vi "1.PROYECTO_FINAL_ESTACIONAMIENTO.vi"() -> ()   [LabVIEW 2025]
uses:
  <vilib>/userDefined/High Color/IMAQdx.ctl
  <vilib>/httpClient/LabVIEWHTTPClient.lvlib
  <vilib>/vision/driver/NI_Vision_Acquisition_Software.lvlib
  <vilib>/vision/NI_Vision_Development_Module.lvlib
panel:
  in  "PAGAR":bool
  out "Total a pagar":string
  out "Tiempo":string
  out "ID TICKET":string
  out "LED1":bool
  out "LED3":bool
  out "LED2":bool
  out "?":string
  out "?":string
  out "LED ticket":bool
  in  "QR_boton":bool
  out "Cámara Estacionamiento":T1(plugin-control)
  out "Camara Qr":T1(plugin-control)
  in  "stop":bool
  out "QR":T1(plugin-control)
  # "ID TICKET"
  # "TIEMPO:"
  # "TOTAL A PAGAR:"
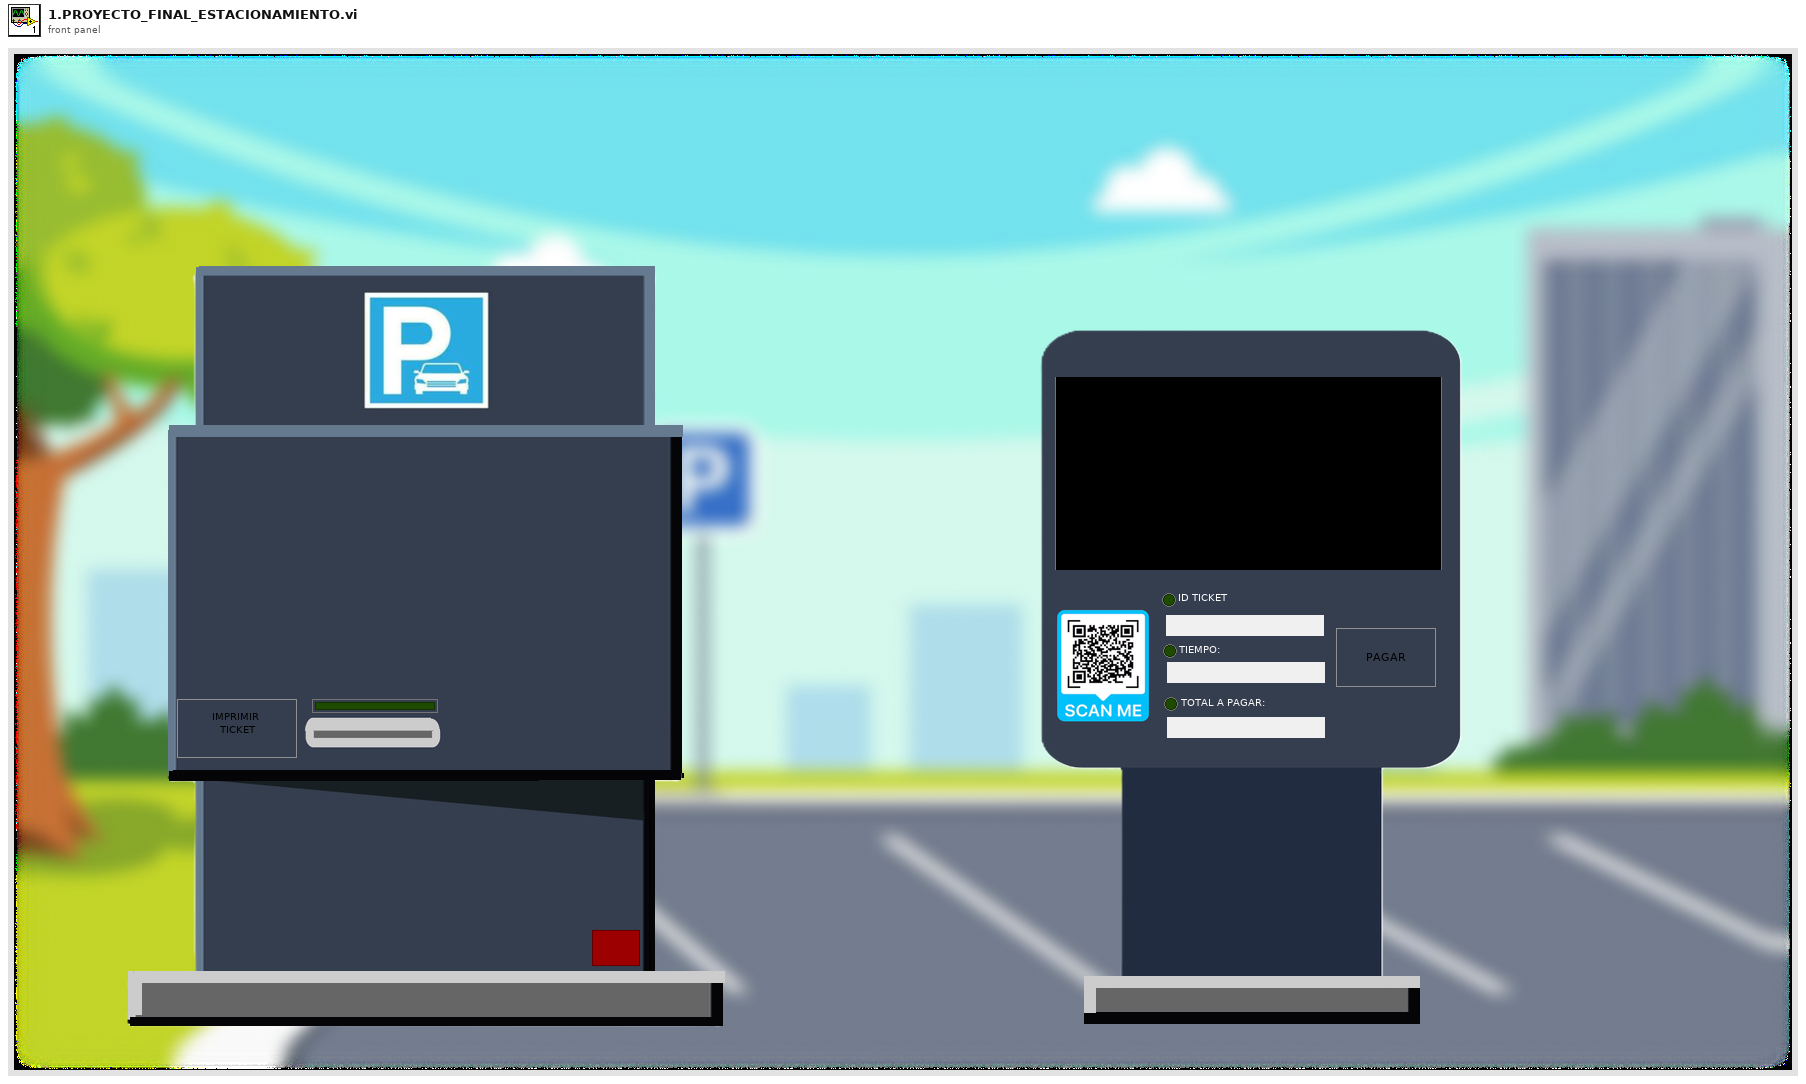
[diagram p1: front panel]
types:
  T1 = typedef "IMAQ Image.ctl" = refnum<image>
  T2 = typedef "Image Type" = u32
  T3 = typedef "IMAQdx.ctl" = refnum<k21>
  T4 = typedef "LabVIEWHTTPClient.lvlib/ClientHandle.ctl" = refnum<k1>
  T5 = typedef "QR Code Report.ctl" = cluster{"Found?":bool, "Data":string, "Bounding Box":cluster{"x":sgl, "y":sgl}[], "Errors Corrected":u32, "Dimensions (Rows/Cols)":u32, "Version":u32, "QR Model":T6, "Stream Mode":T7, "Barcode Polarity":T8, "Mirrored?":bool, "Append Stream Position":u32, "Size of Append Stream":u32, "First EAN-128 ID":i32, "First Alternate Language ID":i32, "Append Stream ID":u32, "Minimum Edge Strength":u32, "Demodulation Mode":T9, "Cell Sample Size":T10, "Cell Filter Mode":T11}
  T6 = typedef "QR Code Model Type.ctl" = i32
  T7 = typedef "QR Code Stream Mode Type.ctl" = i32
  T8 = typedef "Data Matrix Polarity.ctl" = i32
  T9 = typedef "Demodulation Mode.ctl" = i32
  T10 = typedef "Cell Sample Size.ctl" = i32
  T11 = typedef "Cell Filter Mode.ctl" = i32
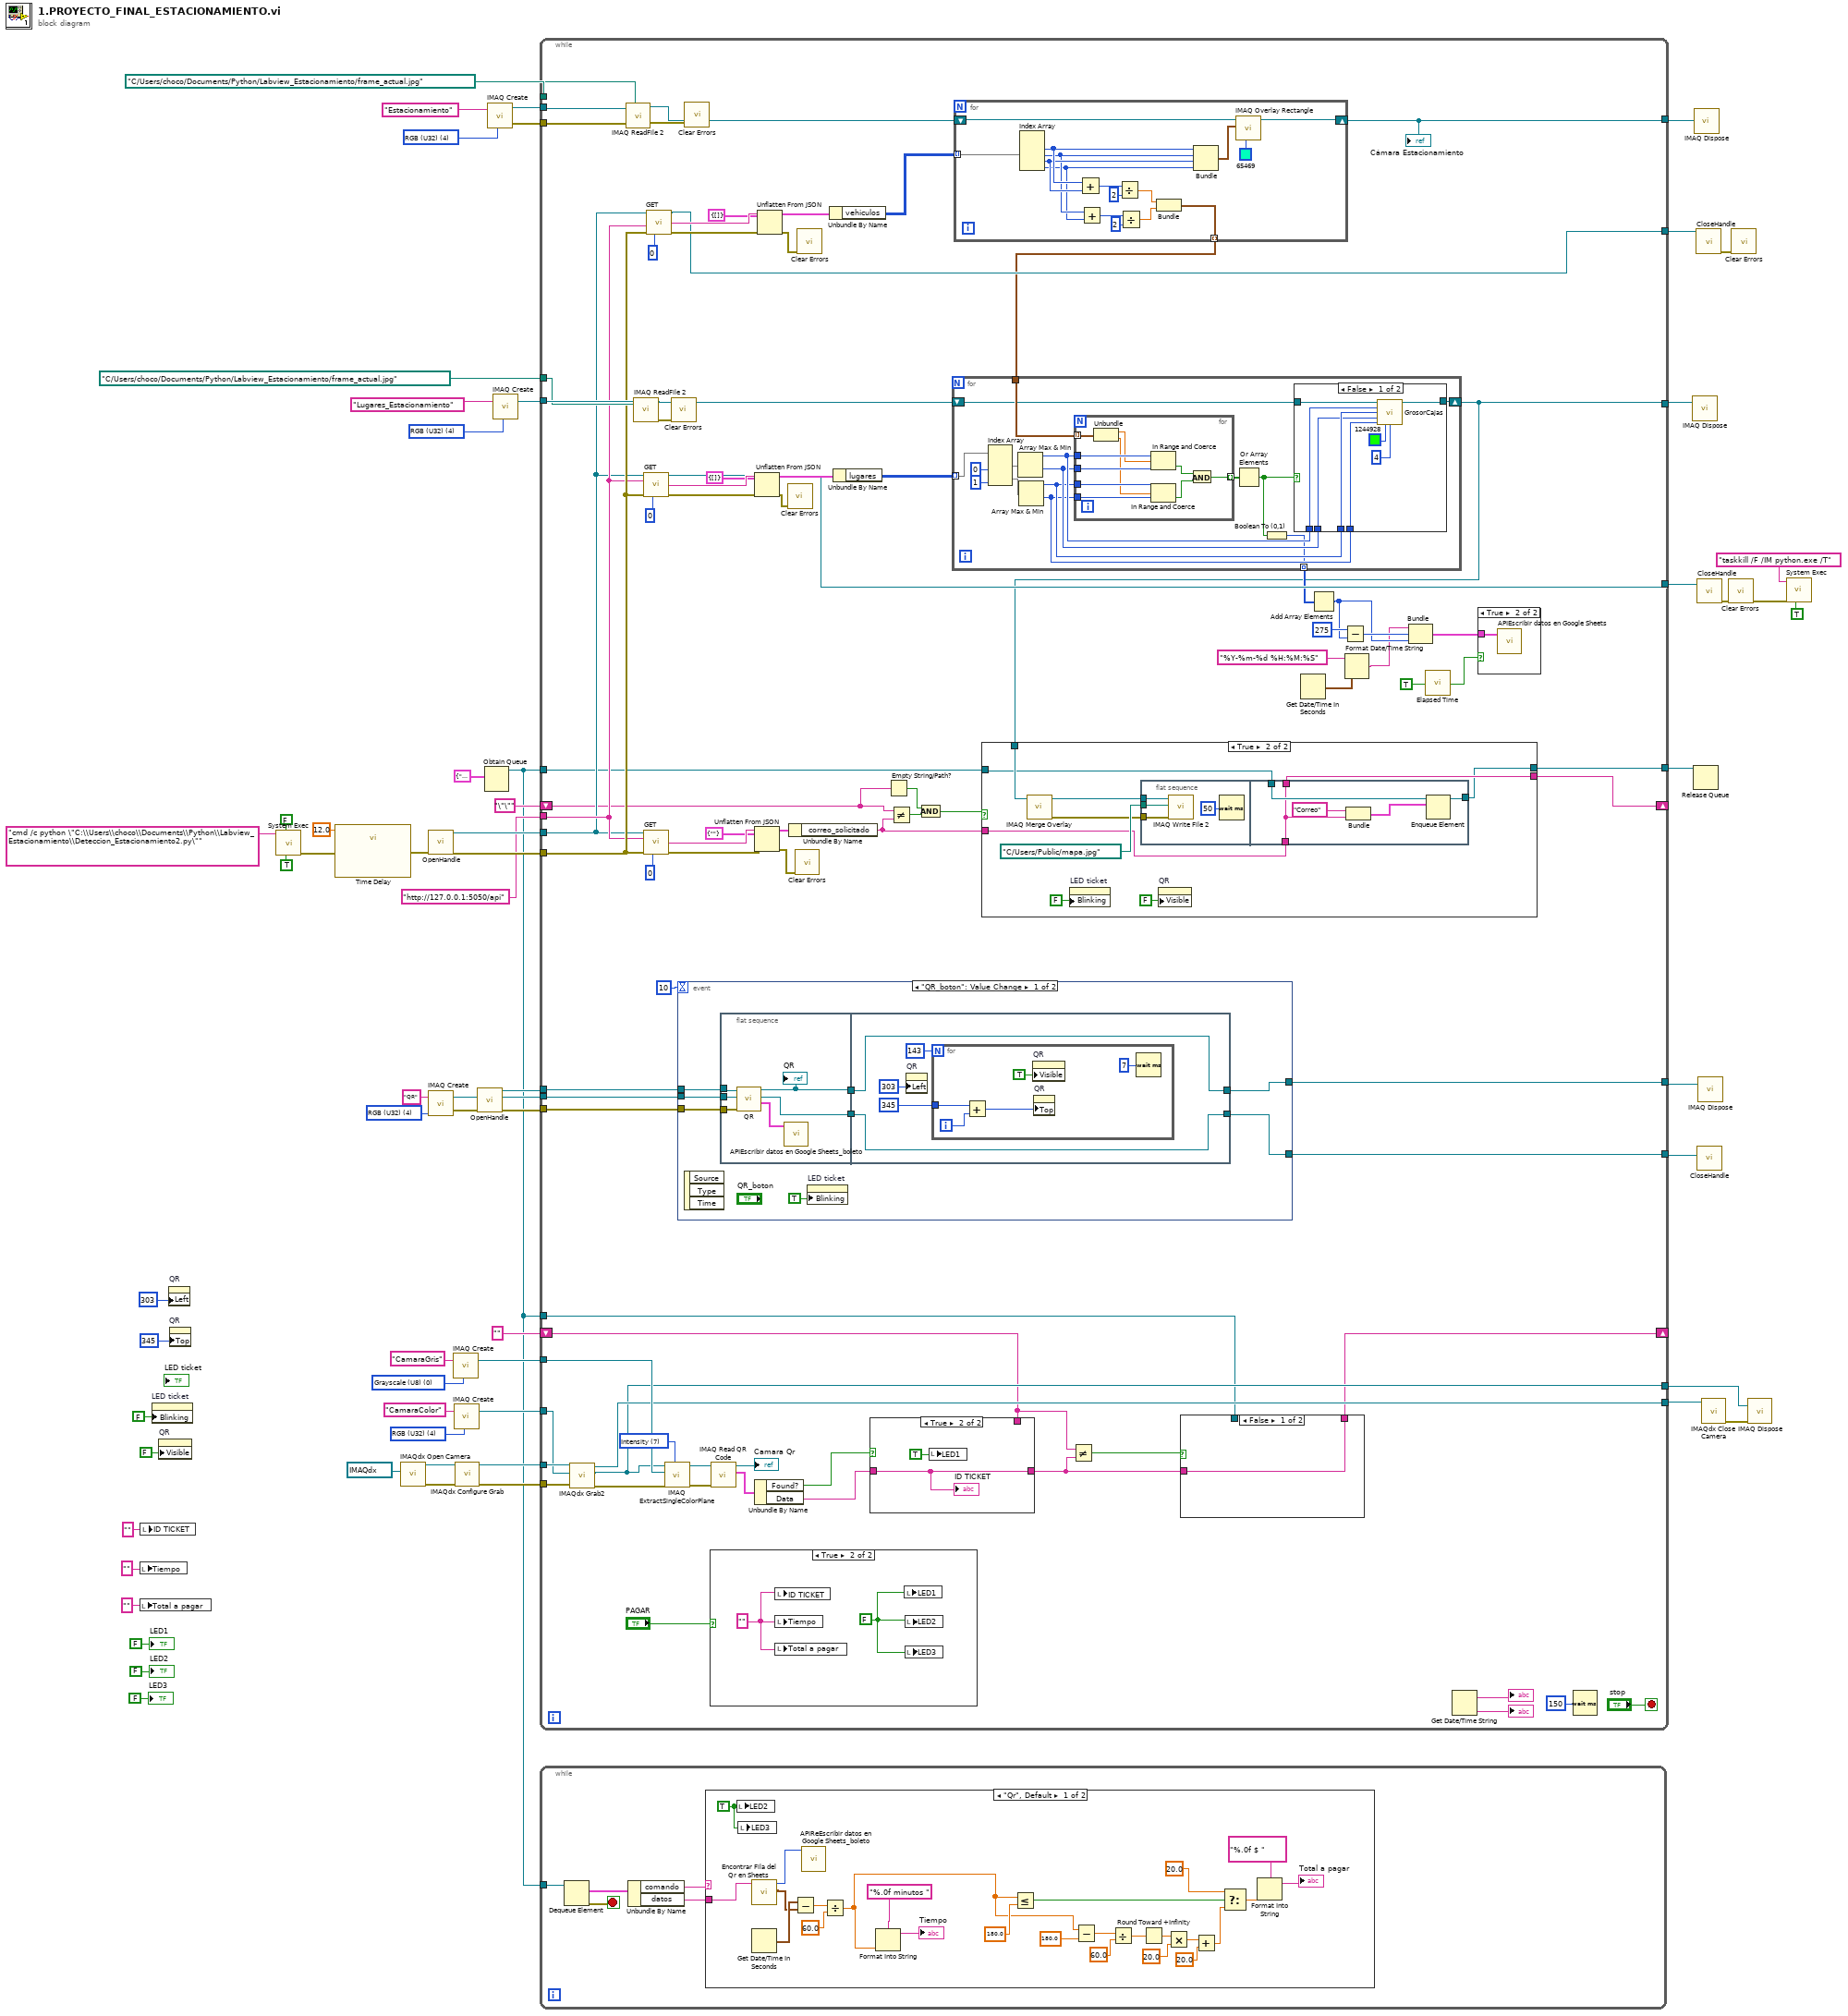
[diagram p0: block diagram]
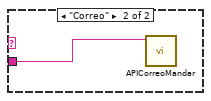
[diagram p2: hidden frame]
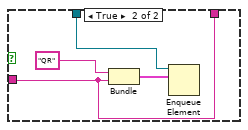
[diagram p4: hidden frame]
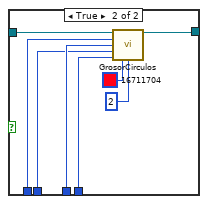
[diagram p7: hidden frame]
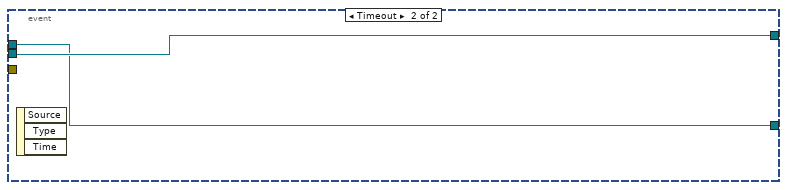
[diagram p9: hidden frame]
diagram:
  w21 = T2 0 items=["Grayscale (U8)", "Grayscale (I16)", "Grayscale (SGL)", "Complex (CSG)", "RGB (U32)", "HSL (U32)", "RGB (U64)", "Grayscale (U16)"] ("Image Type")
  w27 = T2 4 items=["Grayscale (U8)", "Grayscale (I16)", "Grayscale (SGL)", "Complex (CSG)", "RGB (U32)", "HSL (U32)", "RGB (U64)", "Grayscale (U16)"] ("Image Type")
  w38 = T2 4 items=["Grayscale (U8)", "Grayscale (I16)", "Grayscale (SGL)", "Complex (CSG)", "RGB (U32)", "HSL (U32)", "RGB (U64)", "Grayscale (U16)"] ("Image Type")
  w49 = T2 4 items=["Grayscale (U8)", "Grayscale (I16)", "Grayscale (SGL)", "Complex (CSG)", "RGB (U32)", "HSL (U32)", "RGB (U64)", "Grayscale (U16)"] ("Image Type")
  w62 = T2 4 items=["Grayscale (U8)", "Grayscale (I16)", "Grayscale (SGL)", "Complex (CSG)", "RGB (U32)", "HSL (U32)", "RGB (U64)", "Grayscale (U16)"] ("Image Type")
  n1 = local write "Tiempo"("" ("Tiempo")) -> ()
  n2 = local write "Total a pagar"("" ("Total a pagar")) -> ()
  n3 = local write "ID TICKET"("" ("ID TICKET")) -> ()
  n4 = property on="LED ticket" class="Bool (strict)"("Blinking"=FALSE) -> ()  [unwired: 2 in, 2 out]
  n5 = property on="QR" class="ImageControl"("Visible"=FALSE) -> ()  [unwired: 2 in, 2 out]
  n6 = property on="QR" class="ImageControl"("Left"=303 ("Position:Left")) -> ()  [unwired: 2 in, 2 out]
  n7 = property on="QR" class="ImageControl"("Top"=345 ("Position:Top")) -> ()  [unwired: 2 in, 2 out]
  n8 = call <vilib>:"System Exec.vi"("run minimized? (F)"=TRUE, "wait until completion? (T)"=FALSE, "command line"="cmd /c python \"C:\\Users\\choco\\Documents\\Python\\Labview_Estacionamiento\\Deteccion_Estacionamiento2.py\"") -> ("error out"=w58:errorcluster)  [unwired: 5 in, 3 out]
  n9 = call "Time Delay"("error in (no error)"=w58, "Delay Time (s)"=12.0) -> ("error out"=w55:errorcluster)  [unwired: 9 in]
  n10 = call <vilib>:"IMAQdx Open Camera.vi"("Session In"=T3 "cam0") -> ("error out"=w24:errorcluster, "Session Out"=w25:T3)  [unwired: 9 in]
  n11 = call <vilib>:"OpenHandle.vi"("error in (no error)"=w55) -> ("client handle out"=w31:T4, "error out"=w32:errorcluster)  [unwired: 13 in]
  n12 = call "IMAQ Create"("Image Name"="QR", "Image Type"=w49) -> ("New Image"=w48:T1, "error out"=w45:errorcluster)  [unwired: 3 in]
  n13 = call "IMAQ Create"("Image Name"="CamaraGris", "Image Type"=w21) -> ("New Image"=w17:T1)  [unwired: 3 in, 1 out]
  n14 = call "IMAQ Create"("Image Name"="CamaraColor", "Image Type"=w27) -> ("New Image"=w18:T1)  [unwired: 3 in, 1 out]
  n15 = call <vilib>:"IMAQdx Configure Grab.vi"("error in"=w24, "Session In"=w25) -> ("error out"=w19:errorcluster, "Session Out"=w20:T3)  [unwired: 8 in]
  n16 = call <vilib>:"OpenHandle.vi"("error in (no error)"=w45) -> ("client handle out"=w46:T4, "error out"=w44:errorcluster)  [unwired: 13 in]
  n17 = Obtain Queue(element data type=cluster{"comando":string, "datos":string} {"comando"="", "datos"=""}) -> (queue out=w11:refnum<queue>)  [unwired: 4 in, 2 out]
  n18 = call "IMAQ Create"("Image Name"="Estacionamiento", "Image Type"=w62) -> ("New Image"=w61:T1, "error out"=w54:errorcluster)  [unwired: 3 in]
  n19 = call "IMAQ Create"("Image Name"="Lugares_Estacionamiento", "Image Type"=w38) -> ("New Image"=w37:T1)  [unwired: 3 in, 1 out]
  n20 = while {
    tunnel: path "C:/Users/choco/Documents/Python/Labview_Estacionamiento/frame_actual.jpg" ("path to JPEG file") -> [w147]
    tunnel: w61 -> [w148]
    tunnel: w54 -> [w145]
    tunnel: [w142] -> w51
    tunnel: w44 -> [w141]
    tunnel: w48 -> [w140]
    tunnel: [w139] -> w47
    tunnel: w46 -> [w138]
    tunnel: [w128] -> w43
    tunnel: [w122] -> w40
    tunnel: w37 -> [w117]
    tunnel: path "C:/Users/choco/Documents/Python/Labview_Estacionamiento/frame_actual.jpg" ("path to JPEG file 2") -> [w116]
    tunnel: [w114] -> w35
    tunnel: [w94] -> w34
    tunnel: w32 -> [w101]
    tunnel: w31 -> [w99]
    tunnel: "http://127.0.0.1:5050/api" ("url") -> [w100]
    shift-right: [w93] -> _
    shift-left: "\"\"" -> [w92]
    tunnel: w11 -> [w90]
    tunnel: w20 -> [w85]
    tunnel: w19 -> [w84]
    tunnel: w18 -> [w83]
    tunnel: w17 -> [w82]
    tunnel: [w81] -> w16
    tunnel: [w80] -> w15
    tunnel: [w79] -> w14
    shift-right: [w73] -> _
    shift-left: "" -> [w68]
    tunnel: w11 -> [w70]
    stop <- "stop" stop-if-true
    w86 = 7 items=["Red", "Green", "Blue", "Hue", "Saturation", "Luminance", "Value", "Intensity"] ("Color Plane")
    n21 = call <vilib>:"IMAQdx Grab2.vi"("error in"=w84, "Image In"=w83, "Session In"=w85) -> ("error out"=w87:errorcluster, "Image Out"=w80:T1, "Session Out"=w81:T3)  [unwired: 5 in, 1 out]
    n22 = call "IMAQ ReadFile 2"("File Path"=w147, "error in (no error)"=w145, "Image"=w148) -> ("error out"=w146:errorcluster, "Image Out"=w119:T1)  [unwired: 4 in, 3 out]
    n23 = call "IMAQ ReadFile 2"("File Path"=w116, "Image"=w117) -> ("error out"=w118:errorcluster, "Image Out"=w115:T1)  [unwired: 5 in, 3 out]
    n24 = call <vilib>:"GET.vi"("client handle"=w99, "url"=w100, "error in (no error)"=w101, "timeout (10000)"=0) -> ("client handle out"=w122:T4, "body"=w127:string, "error out"=w126:errorcluster)  [unwired: 8 in, 1 out]
    n25 = call <vilib>:"GET.vi"("client handle"=w99, "url"=w100, "error in (no error)"=w101, "timeout (10000)"=0) -> ("body"=w105:string, "error out"=w104:errorcluster)  [unwired: 8 in, 2 out]
    n26 = call <vilib>:"GET.vi"("client handle"=w99, "url"=w100, "error in (no error)"=w101, "timeout (10000)"=0) -> ("client handle out"=w128:T4, "body"=w136:string, "error out"=w135:errorcluster)  [unwired: 8 in, 1 out]
    n27 = call "IMAQ ExtractSingleColorPlane"("Color Plane"=w86, "error in (no error)"=w87, "Image Dst"=w82, "Image Src"=w80) -> ("error out"=w76:errorcluster, "Image Dst Out"=w77:T1)  [unwired: 6 in]
    n28 = call <vilib>:"Clear Errors.vi"("error in (no error)"=w118) -> ()  [unwired: 5 in, 2 out]
    n29 = event shown="[0] \"QR_boton\": Value Change" {
      selector: _ -> [_ _]
      dyn-events: _ -> [_ _]
      timeout: 10 -> [_ _]
      tunnel: [w242 w264] -> w142
      tunnel: w141 -> [w246 _]
      tunnel: w140 -> [w245 w264]
      tunnel: [w243 w263] -> w139
      tunnel: w138 -> [w244 w263]
      event "QR_boton": Value Change {
        n30 = event-data() -> ()  [unwired: 1 in, 3 out]
        n31 = flat-sequence {
          tunnel: w246 -> [w252]
          tunnel: w245 -> [w251]
          tunnel: w244 -> [w250]
          tunnel: [w249] -> w241
          tunnel: [w248] -> w240
          tunnel: [w257] -> w242
          tunnel: [w256] -> w243
          tunnel: w241 -> [w256]
          tunnel: w240 -> [w257]
          frame #0 {
            n32 = call "QR.vi"("error in (no error)"=w252, "Image"=w251, "client handle"=w250) -> ("value"=w247:cluster{"id":string, "hora_entrada":string}, "client handle out"=w249:T4, "QR Imagen"=w248:T1)  [unwired: 6 in]
            "QR" <- w248
            n33 = call "APIEscribir datos en Google Sheets_boleto.vi"("Cluster"=w247) -> ()  [unwired: 10 in]
          }
          frame #1 {
            n34 = property on="QR" class="ImageControl"("Left"=303 ("Position:Left")) -> ()  [unwired: 2 in, 2 out]
            n35 = for {
              N: 143 -> [_]
              tunnel: 345 ("Position:Top") -> [w259]
              i -> [w262]
              n36 = Add(x=w259, y=w262) -> (x+y=w261:i32)
              n37 = property on="QR" class="ImageControl"("Visible"=TRUE) -> ()  [unwired: 2 in, 2 out]
              n38 = property on="QR" class="ImageControl"("Top"=w261) -> ()  [unwired: 2 in, 2 out]
              n39 = Wait (ms)(milliseconds to wait=u32 7) -> ()  [unwired: 1 out]
            }
          }
        }
        n40 = property on="LED ticket" class="Bool (strict)"("Blinking"=TRUE) -> ()  [unwired: 2 in, 2 out]
      }
      event Timeout {
        n41 = event-data() -> ()  [unwired: 1 in, 3 out]
      }
    }
    n42 = call <vilib>:"Clear Errors.vi"("error in (no error)"=w146) -> ()  [unwired: 5 in, 2 out]
    n43 = case shown="True" "PAGAR" {
      frame False {
      }
      frame True {
        w150 = FALSE
        w151 = "" ("ID TICKET")
        n44 = local write "ID TICKET"(w151) -> ()
        n45 = local write "Tiempo"(w151) -> ()
        n46 = local write "Total a pagar"(w151) -> ()
        n47 = local write "LED1"(w150) -> ()
        n48 = local write "LED2"(w150) -> ()
        n49 = local write "LED3"(w150) -> ()
      }
    }
    n50 = call "IMAQ Read QR Code"("error in (no error)"=w76, "Image"=w77) -> ("QR Code Report"=w78:T5, "Image (duplicate)"=→"Camara Qr":T1)  [unwired: 6 in, 2 out]
    n51 = Unbundle By Name(w78) -> ("Found?"=w75:bool, "Data"=w74:string)
    n52 = Unflatten From JSON(JSON string=w127, type and defaults=cluster{"lugares":i32[][][]} {"lugares"=[]}, error in (no error)=w126) -> (value=w123:cluster{"lugares":i32[][][]}, error out=w71:errorcluster)  [unwired: 4 in]
    n53 = Unflatten From JSON(JSON string=w105, type and defaults=cluster{"correo_solicitado":string} {"correo_solicitado"=""}, error in (no error)=w104) -> (value=w98:cluster{"correo_solicitado":string}, error out=w69:errorcluster)  [unwired: 4 in]
    n54 = Unflatten From JSON(JSON string=w136, type and defaults=cluster{"vehiculos":i32[][]} {"vehiculos"=[]}, error in (no error)=w135) -> (value=w132:cluster{"vehiculos":i32[][]}, error out=w72:errorcluster)  [unwired: 4 in]
    n55 = call <vilib>:"Clear Errors.vi"("error in (no error)"=w71) -> ()  [unwired: 5 in, 2 out]
    n56 = Unbundle By Name(w98) -> ("correo_solicitado"=w91:string)
    n57 = call <vilib>:"Clear Errors.vi"("error in (no error)"=w69) -> ()  [unwired: 5 in, 2 out]
    n58 = call <vilib>:"Clear Errors.vi"("error in (no error)"=w72) -> ()  [unwired: 5 in, 2 out]
    n59 = Unbundle By Name(w132) -> ("vehiculos"=w131:i32[][])
    n60 = Unbundle By Name(w123) -> ("lugares"=w121:i32[][][])
    n61 = case shown="True" w75 {
      tunnel: w74 -> [_ w159]
      tunnel: [w157 w159] -> w67
      tunnel: w68 -> [w157 _]
      frame False {
      }
      frame True {
        n62 = local write "LED1"(TRUE ("LED1")) -> ()
        "ID TICKET" <- w159
      }
    }
    n63 = Empty String/Path?(string/path=w92) -> (empty?=w96:bool)
    n64 = Not Equal?(x=w92, y=w91) -> (x != y?=w97:bool)
    n65 = And(x=w96, y=w97) -> (x .and. y?=w95:bool)
    n66 = for {
      tunnel: w131 -> [w238] mode=indexing
      shift-right: [w236] -> w114
      shift-left: w119 -> [w234]
      tunnel: [w223] -> w120 mode=indexing
      n67 = Index Array(array=w238) -> (element #1=w233:i32, element #2=w227:i32, element #3=w232:i32, element #4=w226:i32)  [unwired: 4 in]
      n68 = Add(x=w233, y=w232) -> (x+y=w231:i32)
      n69 = Add(x=w227, y=w226) -> (x+y=w229:i32)
      n70 = Divide(x=w231, y=2) -> (x/y=w225:dbl)
      n71 = Divide(x=w229, y=2) -> (x/y=w224:dbl)
      n72 = Bundle(w225, w224) -> (w223:cluster{dbl, dbl})  [unwired: 1 in]
      n73 = Bundle(w233, w227, w232, w226) -> (w237:cluster{i32, i32, i32, i32})  [unwired: 1 in]
      n74 = call "IMAQ Overlay Rectangle"("Color"=u32 65469, "Rectangle"=w237, "Image"=w234) -> ("Image Out"=w236:T1)  [unwired: 7 in, 1 out]
    }
    "Cámara Estacionamiento" <- w114
    n75 = for {
      tunnel: w121 -> [w195] mode=indexing
      tunnel: w120 -> [w190]
      shift-right: [w183] -> w94
      shift-left: w115 -> [w184]
      tunnel: [w181] -> w112 mode=indexing
      n76 = Index Array(array=w195, index (col) #1=0 ("disabled index (col)"), index (col) #2=1 ("index (col)")) -> (element #1=w192:i32[], element #2=w191:i32[])  [unwired: 2 in]
      n77 = Array Max & Min(array=w192) -> (max value=w188:i32, min value=w187:i32)  [unwired: 2 out]
      n78 = Array Max & Min(array=w191) -> (max value=w186:i32, min value=w185:i32)  [unwired: 2 out]
      n79 = for {
        tunnel: w188 -> [w221]
        tunnel: w187 -> [w220]
        tunnel: w186 -> [w219]
        tunnel: w185 -> [w218]
        tunnel: w190 -> [w217] mode=indexing
        tunnel: [w212] -> w189 mode=indexing
        n80 = Unbundle(w217) -> (w216:dbl, w215:dbl)
        n81 = In Range and Coerce(upper limit=w221, x=w216, lower limit=w220) -> (In Range?=w214:bool)  [unwired: 1 out]
        n82 = In Range and Coerce(upper limit=w219, x=w215, lower limit=w218) -> (In Range?=w213:bool)  [unwired: 1 out]
        n83 = And(x=w214, y=w213) -> (x .and. y?=w212:bool)
      }
      n84 = Or Array Elements(Boolean array=w189) -> (logical OR=w182:bool)
      n85 = Boolean To (0,1)(Boolean=w182) -> (0, 1=w181:i16)
      n86 = case shown="False" w182 {
        tunnel: w188 -> [w203 w211]
        tunnel: w187 -> [w201 w209]
        tunnel: w186 -> [w202 w210]
        tunnel: w185 -> [w200 w208]
        tunnel: w184 -> [w199 w207]
        tunnel: [w196 w204] -> w183
        frame False {
          n87 = call "GrosorCajas.vi"("Imagen"=w199, "x_min"=w203, "y_min"=w202, "x_max"=w201, "y_max"=w200, "Color"=u32 1244928, "Grosor"=4) -> ("Imagen salida"=w196:T1)  [unwired: 8 in]
        }
        frame True {
          n88 = call "GrosorCirculos.vi"("Imagen"=w207, "x_min"=w211, "y_min"=w210, "x_max"=w209, "y_max"=w208, "Color"=u32 16711704, "Grosor"=2) -> ("Imagen salida"=w204:T1)  [unwired: 8 in]
        }
      }
    }
    n89 = case shown="True" w95 {
      tunnel: w94 -> [_ w171]
      tunnel: w91 -> [w161 w167]
      tunnel: [w161 w166] -> w93
      tunnel: w90 -> [w160 w165]
      tunnel: [w160 w164] -> w79
      frame False {
      }
      frame True {
        n90 = call "IMAQ Merge Overlay"("Image Src"=w171) -> ("error out"=w168:errorcluster, "Image Dst Out"=w170:T1)  [unwired: 9 in]
        n91 = property on="LED ticket" class="Bool (strict)"("Blinking"=FALSE) -> ()  [unwired: 2 in, 2 out]
        n92 = flat-sequence {
          tunnel: w170 -> [w175]
          tunnel: path "C:/Users/Public/mapa.jpg" ("file (use dialog)") -> [w174]
          tunnel: w168 -> [w173]
          tunnel: w167 -> [w178]
          tunnel: [w178] -> w166
          tunnel: w165 -> [w179]
          tunnel: [w180] -> w164
          frame #0 {
            n93 = call-poly "IMAQ Write File 2"("error in (no error)"=w173, "File Path"=w174, "Image"=w175) -> ()  [unwired: 7 in, 2 out]
            n94 = Wait (ms)(milliseconds to wait=u32 50) -> ()  [unwired: 1 out]
          }
          frame #1 {
            n95 = Bundle("Correo", "correo_solicitado"=w178) -> (w176:cluster{string, "correo_solicitado":string})  [unwired: 1 in]
            n96 = Enqueue Element(queue=w179, element=w176) -> (queue out=w180:refnum<queue>)  [unwired: 2 in, 2 out]
          }
        }
        n97 = property on="QR" class="ImageControl"("Visible"=FALSE) -> ()  [unwired: 2 in, 2 out]
      }
    }
    n98 = Not Equal?(x=w68, y=w67) -> (x != y?=w66:bool)
    n99 = case shown="False" w66 {
      tunnel: [w152 w153] -> w73
      tunnel: w67 -> [w152 w153]
      tunnel: w70 -> [_ w154]
      frame False {
      }
      frame True {
        n100 = Bundle("QR", "Data"=w153) -> (w155:cluster{string, "Data":string})  [unwired: 1 in]
        n101 = Enqueue Element(queue=w154, element=w155) -> ()  [unwired: 2 in, 3 out]
      }
    }
    n102 = Get Date/Time In Seconds() -> (seconds since 1Jan1904=w109:timestamp)
    n103 = Add Array Elements(numeric array=w112) -> (sum=w110:i16)
    n104 = Subtract(x=275, y=w110) -> (x-y=w111:i32)
    n105 = Format Date/Time String(time format string (%c)="%Y-%m-%d %H:%M:%S", seconds (now)=w109) -> (date/time string=w107:string)  [unwired: 1 in]
    n106 = Bundle("date/time string"=w107, w111, w110) -> (w106:cluster{"date/time string":string, i32, i16})  [unwired: 1 in]
    n107 = call "Elapsed Time"("Auto Reset"=TRUE) -> ("Time has Elapsed"=w129:bool)  [unwired: 11 in, 7 out]
    n108 = Get Date/Time String() -> (date string=→"?":string, time string=→"?":string)  [unwired: 3 in]
    n109 = case shown="True" w129 {
      tunnel: w106 -> [_ w222]
      frame False {
      }
      frame True {
        n110 = call "APIEscribir datos en Google Sheets.vi"("Cluster"=w222) -> ()  [unwired: 10 in]
      }
    }
    n111 = Wait (ms)(milliseconds to wait=u32 150) -> ()  [unwired: 1 out]
  }
  n112 = while {
    tunnel: w11 -> [w269]
    stop <- w268 stop-if-true
    n113 = Dequeue Element(queue=w269) -> (element=w267:cluster{"comando":string, "datos":string}, error out=w268:errorcluster)  [unwired: 2 in, 2 out]
    n114 = Unbundle By Name(w267) -> ("comando"=w266:string, "datos"=w265:string)
    n115 = case shown="\"Qr\", Default" w266 {
      tunnel: w265 -> [w294 w295]
      frame "Qr", Default {
        w271 = TRUE ("LED2")
        n116 = local write "LED2"(w271) -> ()
        n117 = local write "LED3"(w271) -> ()
        n118 = call "Encontrar Fila del Qr en Sheets.vi"("QR"=w294) -> ("hora_entrada"=w291:timestamp, "indice del QR"=w293:i32)  [unwired: 9 in]
        n119 = Get Date/Time In Seconds() -> (seconds since 1Jan1904=w292:timestamp)
        n120 = Subtract(x=w292, y=w291) -> (x-y=w290:dbl)
        n121 = call "APIReEscribir datos en Google Sheets_boleto.vi"("fila"=w293) -> ()  [unwired: 10 in]
        n122 = Divide(x=w290, y=60.0) -> (x/y=w275:dbl)
        n123 = Format Into String(format string="%.0f minutos ", w275) -> (resulting string=→"Tiempo":string)  [unwired: 2 in, 1 out]
        n124 = Less Or Equal?(x=w275, y=180.0) -> (x <= y?=w287:bool)
        n125 = Subtract(x=w275, y=180.0 ("t")) -> (x-y=w284:dbl)
        n126 = Divide(x=w284, y=60.0) -> (x/y=w282:dbl)
        n127 = Round Toward +Infinity(x=w282) -> (ceil(x): smallest int >= x=w281:dbl)
        n128 = Multiply(x=w281, y=20.0) -> (x*y=w279:dbl)
        n129 = Add(x=w279, y=20.0) -> (x+y=w277:dbl)
        n130 = Select(t=20.0, s=w287, f=w277) -> (s? t:f=w273:dbl)
        n131 = Format Into String(format string="%.0f $ ", w273) -> (resulting string=→"Total a pagar":string)  [unwired: 2 in, 1 out]
      }
      frame "Correo" {
        n132 = call "APICorreoMandar.vi"("Correo"=w295) -> ()  [unwired: 9 in]
      }
    }
  }
  n133 = call "IMAQ Dispose"("Image"=w34) -> ()  [unwired: 5 in, 1 out]
  n134 = Release Queue(queue=w14) -> ()  [unwired: 2 in, 3 out]
  n135 = call "IMAQ Dispose"("Image"=w35) -> ()  [unwired: 5 in, 1 out]
  n136 = call <vilib>:"CloseHandle.vi"("client handle"=w43) -> ("error out"=w42:errorcluster)  [unwired: 14 in]
  n137 = call <vilib>:"CloseHandle.vi"("client handle"=w40) -> ("error out"=w41:errorcluster)  [unwired: 14 in]
  n138 = call <vilib>:"CloseHandle.vi"("client handle"=w47) -> ()  [unwired: 14 in, 1 out]
  n139 = call "IMAQ Dispose"("Image"=w51) -> ()  [unwired: 5 in, 1 out]
  n140 = call <vilib>:"IMAQdx Close Camera.vi"("Session In"=w16) -> ("error out"=w23:errorcluster)  [unwired: 10 in]
  n141 = call <vilib>:"Clear Errors.vi"("error in (no error)"=w41) -> ("error out"=w33:errorcluster)  [unwired: 5 in, 1 out]
  n142 = call <vilib>:"Clear Errors.vi"("error in (no error)"=w42) -> ()  [unwired: 5 in, 2 out]
  n143 = call "IMAQ Dispose"("Image"=w15, "error in (no error)"=w23) -> ()  [unwired: 4 in, 1 out]
  n144 = call <vilib>:"System Exec.vi"("run minimized? (F)"=TRUE, "error in (no error)"=w33, "command line"="taskkill /F /IM python.exe /T") -> ()  [unwired: 5 in, 4 out]
  "LED2" <- FALSE
  "LED3" <- FALSE
  "LED1" <- FALSE
